vi "TotalRecall_Reload.vi"() -> (0 "gap":i32, 1 "invalid":i32, 2 "valid":i32, 3 "error out":errorcluster)   [LabVIEW 2009]
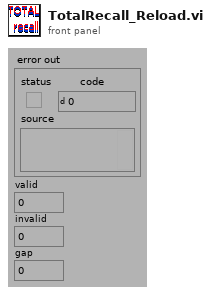
[diagram p1: front panel]
types:
  T1 = typedef "FIFOSettings_BH.ctt" = cluster{"Measurement":cluster{"Binning (ms)":sgl, "External Trigger Condition":u16, "Stop Condition:":u16, "Stop Count":dbl, "Buffer Size (Photons)":u16, "No of Channels":u16, "Ext Latch Delay":i16}, "ADC":cluster{"Module":u16, "ADC Resolution":i32, "Dither Range":i16, "Count Increment":i16, "Macro Time Clock":i16}, "SYNC":cluster{"SYNC ZC Level (mV)":sgl, "SYNC Freq Divider":i16, "SYNC Holdoff (ns)":sgl, "SYNC Threshold (mV)":sgl}, "TAC":cluster{"TAC Range (ns)":sgl, "TAC Gain":i16, "TAC Offset (%)":sgl, "TAC Limit Low (%)":sgl, "TAC Limit High (%)":sgl}, "CFD":cluster{"CFD Limit Low (mV)":sgl, "CFD Limit High (mV)":sgl, "CFD ZC Level (mV)":sgl, "CFD Holdoff (ns)":sgl}}
  T2 = cluster{"router":u8[], "macro times":dbl[], "micro times":u16[], "invalid":dbl[], "gap":dbl[]}
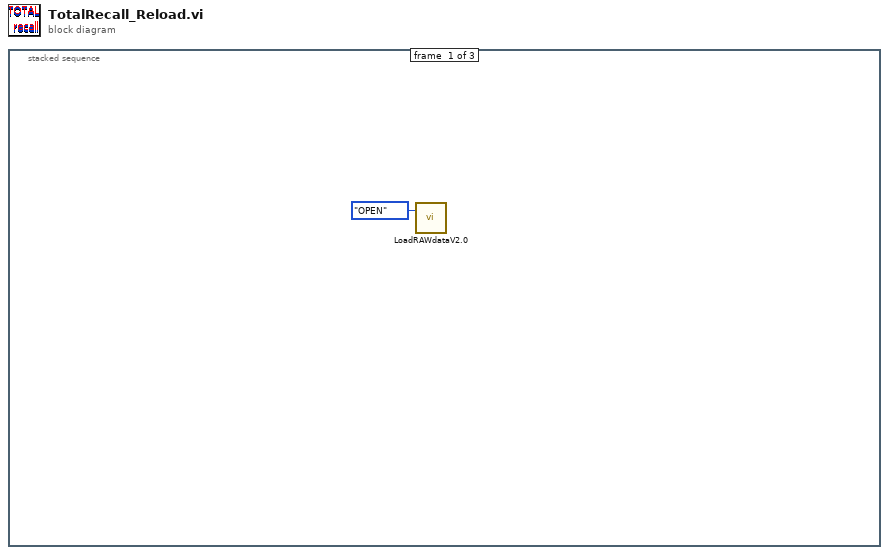
[diagram p0: block diagram]
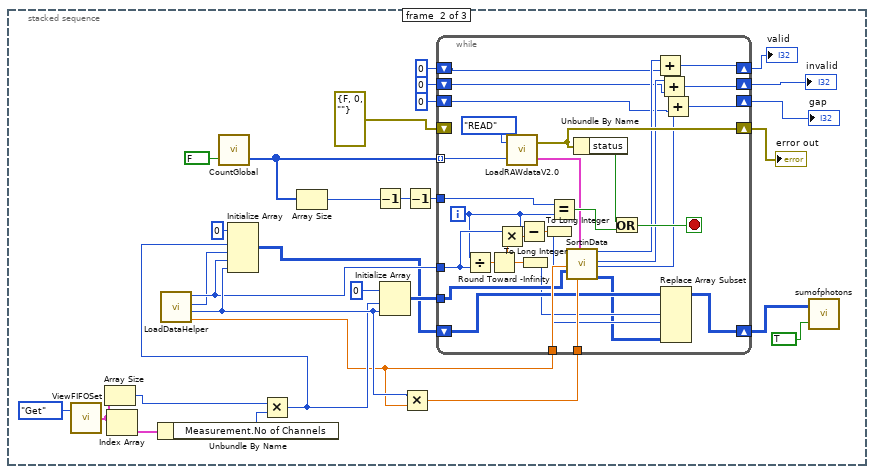
[diagram p2: hidden frame]
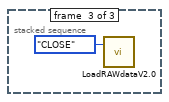
[diagram p3: hidden frame]
diagram:
  n1 = stacked-sequence {
    frame #0 {
      n2 = call "LoadRAWdataV2.0.vi"("action"=enum16{"OPEN", "READ", "CLOSE"}."OPEN" ("Enum")) -> ()  [unwired: 1 in, 2 out]
    }
    frame #1 {
      n3 = call "ViewFIFOSet.vi"("Enum"=enum16{"Display", "change", "Get", "Set"}."Get") -> ("FIFO Settings (Array)"=w6:T1[])  [unwired: 1 in]
      n4 = Array Size(array=w6) -> (size(s)=w5:i32)
      n5 = Index Array(array=w6) -> (element=w7:T1)  [unwired: 1 in]
      n6 = Unbundle By Name(w7) -> ("Measurement.No of Channels"=w4:u16)
      n7 = call "LoadDataHelper.vi"() -> ("Time Resolution [ms/pixel]"=w2:dbl, "pixel per line"=w14:u32, "planes"=w11:u32, "lines"=w13:u32)  [unwired: 7 in, 1 out]
      n8 = call "CountGlobal.vi"("changed?"=FALSE) -> ("count out"=w27:i32[])  [unwired: 2 in]
      n9 = Multiply(x=w5, y=w4) -> (x*y=w3:i32)
      n10 = Initialize Array(u32 0, w3, w11, w13, w14) -> (w10:u32[][][][])
      n11 = Array Size(array=w27) -> (size(s)=w17:i32)
      n12 = Decrement(x=w17) -> (x-1=w26:i32)
      n13 = Initialize Array(u32 0 ("element"), w3, w14) -> (w15:u32[][])
      n14 = Multiply(x=w14, y=w2) -> (x*y=w24:dbl)
      n15 = Decrement(x=w26) -> (x-1=w25:i32)
      n16 = while {
        tunnel: w2 -> [w58]
        tunnel: w27 -> [w44] mode=indexing
        shift-right: [w62] -> w28
        shift-left: errorcluster {"status"=FALSE, "code"=0, "source"=""} ("error out") -> [_]
        tunnel: w25 -> [w57]
        tunnel: w24 -> [w54]
        shift-right: [w50] -> w20
        shift-left: 0 -> [w47]
        shift-right: [w49] -> w19
        shift-left: 0 -> [w46]
        shift-right: [w48] -> w18
        shift-left: 0 -> [w45]
        tunnel: w15 -> [w36]
        tunnel: w13 -> [w41]
        shift-right: [w35] -> w9
        shift-left: w10 -> [w37]
        i -> [w39]
        stop <- w59 stop-if-true
        n17 = Divide(x=w39, y=w41) -> (x/y=w43:dbl)
        n18 = Round Toward -Infinity(1:w43) -> (0:w42:dbl)
        n19 = Multiply(x=w41, y=w42) -> (x*y=w38:dbl)
        n20 = call "LoadRAWdataV2.0.vi"("pos offset (0)"=w44, "action"=enum16{"OPEN", "READ", "CLOSE"}."READ" ("Enum")) -> ("RAW data"=w55:T2, "error out"=w62:errorcluster)
        n21 = Subtract(x=w39, y=w38) -> (x-y=w40:dbl)
        n22 = To Long Integer(number=w42) -> (32bit integer=w34:i32)
        n23 = To Long Integer(number=w40) -> (32bit integer=w33:i32)
        n24 = Equal?(x=w57, y=w39) -> (x = y?=w61:bool)
        n25 = call "SortinData.vi"("binning"=w58, "Array sop"=w36, "rawdata"=w55, "MAT trace/retrace"=w54) -> ("valid"=w53:i32, "invalid"=w52:i32, "gap"=w51:i32, "Array sop 2"=w32:u32[][])  [unwired: 11 in, 1 out]
        n26 = Unbundle By Name(w62) -> ("status"=w60:bool)
        n27 = Or(x=w60, y=w61) -> (x .or. y?=w59:bool)
        n28 = Add(x=w53, y=w47) -> (x+y=w50:i32)
        n29 = Add(x=w52, y=w46) -> (x+y=w49:i32)
        n30 = Replace Array Subset(array=w37, new element=w32, index (dim 1)=w34, index (dim 2)=w33) -> (w35:u32[][][][])  [unwired: 2 in]
        n31 = Add(x=w51, y=w45) -> (x+y=w48:i32)
      }
      "error out" <- w28
      "valid" <- w20
      "invalid" <- w19
      "gap" <- w18
      n32 = call "sumofphotons.vi"("s"=TRUE, "sum of photons"=w9) -> ()  [unwired: 1 out]
    }
    frame #2 {
      n33 = call "LoadRAWdataV2.0.vi"("action"=enum16{"OPEN", "READ", "CLOSE"}."CLOSE" ("Enum")) -> ()  [unwired: 1 in, 2 out]
    }
  }
